vi "Receiver_Example_Img - Copy (2).vi"() -> ()   [LabVIEW 2018]
uses:
  <vilib>/picture/picture.llb/imagedata.ctl
panel:
  in  "path to BMP file":path=path "D:/Thesis Pak Pri/pict.bmp"
  out "Constellation Diagram Receiver":cdb[](graph)
  out "0, 2":i16[][](array[numeric])
  out "1-bit pixmap   2":bool[][](array[boolean])
  out "new picture 2":picture
  out "image data 2":T1
  in  "Image File Reference":path=path "D:/Thesis Pak Pri/boo.bmp"
  out "Array":i32[](array[numeric])
  out "x/y 3":dbl
  out "size bit output":i32
  out "BER":dbl
  out "Numeric":i32
  out "bit output":i32[][](array[numeric])
  out "output diterima":bool[][](array[boolean])
  out "Output Image":picture
  in  "Width":i32=256
  in  "Height":i32=256
  out "x/y":dbl
  out "x > y?":bool
  out "size(s)":i32
  out "bit received":i8[](array[numeric])
  in  "Bit length (set)":i32=3600
  out "sisa bagi":i32
  out "hasil bagi":i32
  out "iterasi":i32
  in  "Modulation parameter":T2
  out "created new?":bool
  out "SIG valid?":bool
  in  "stop":bool
  out "USRP CoercedParamters":T3={"coerced IQ rate"=100000.0, "coerced carrier frequency"=100000.0, "coerced gain"=0.0} {"coerced gain" format="%#_6f"; "coerced carrier frequency" format="%#_6p"; "coerced IQ rate" format="%#_6p"}
  out "error out":errorcluster
  in  "Trigger level":dbl=0.005 format="%f"
  in  "error in (no error)":errorcluster
  in  "USRP ControledParameters":T4={"active antenna"="RX1", "gain"=0.0, "carrier frequency"=915000000.0, "IQ rate"=1000000.0} {"IQ rate" format="%#_6p"; "carrier frequency" format="%#_6p"; "gain" format="%#_6f"}
  in  "device names":refnum<k15>="192.168.10.4"
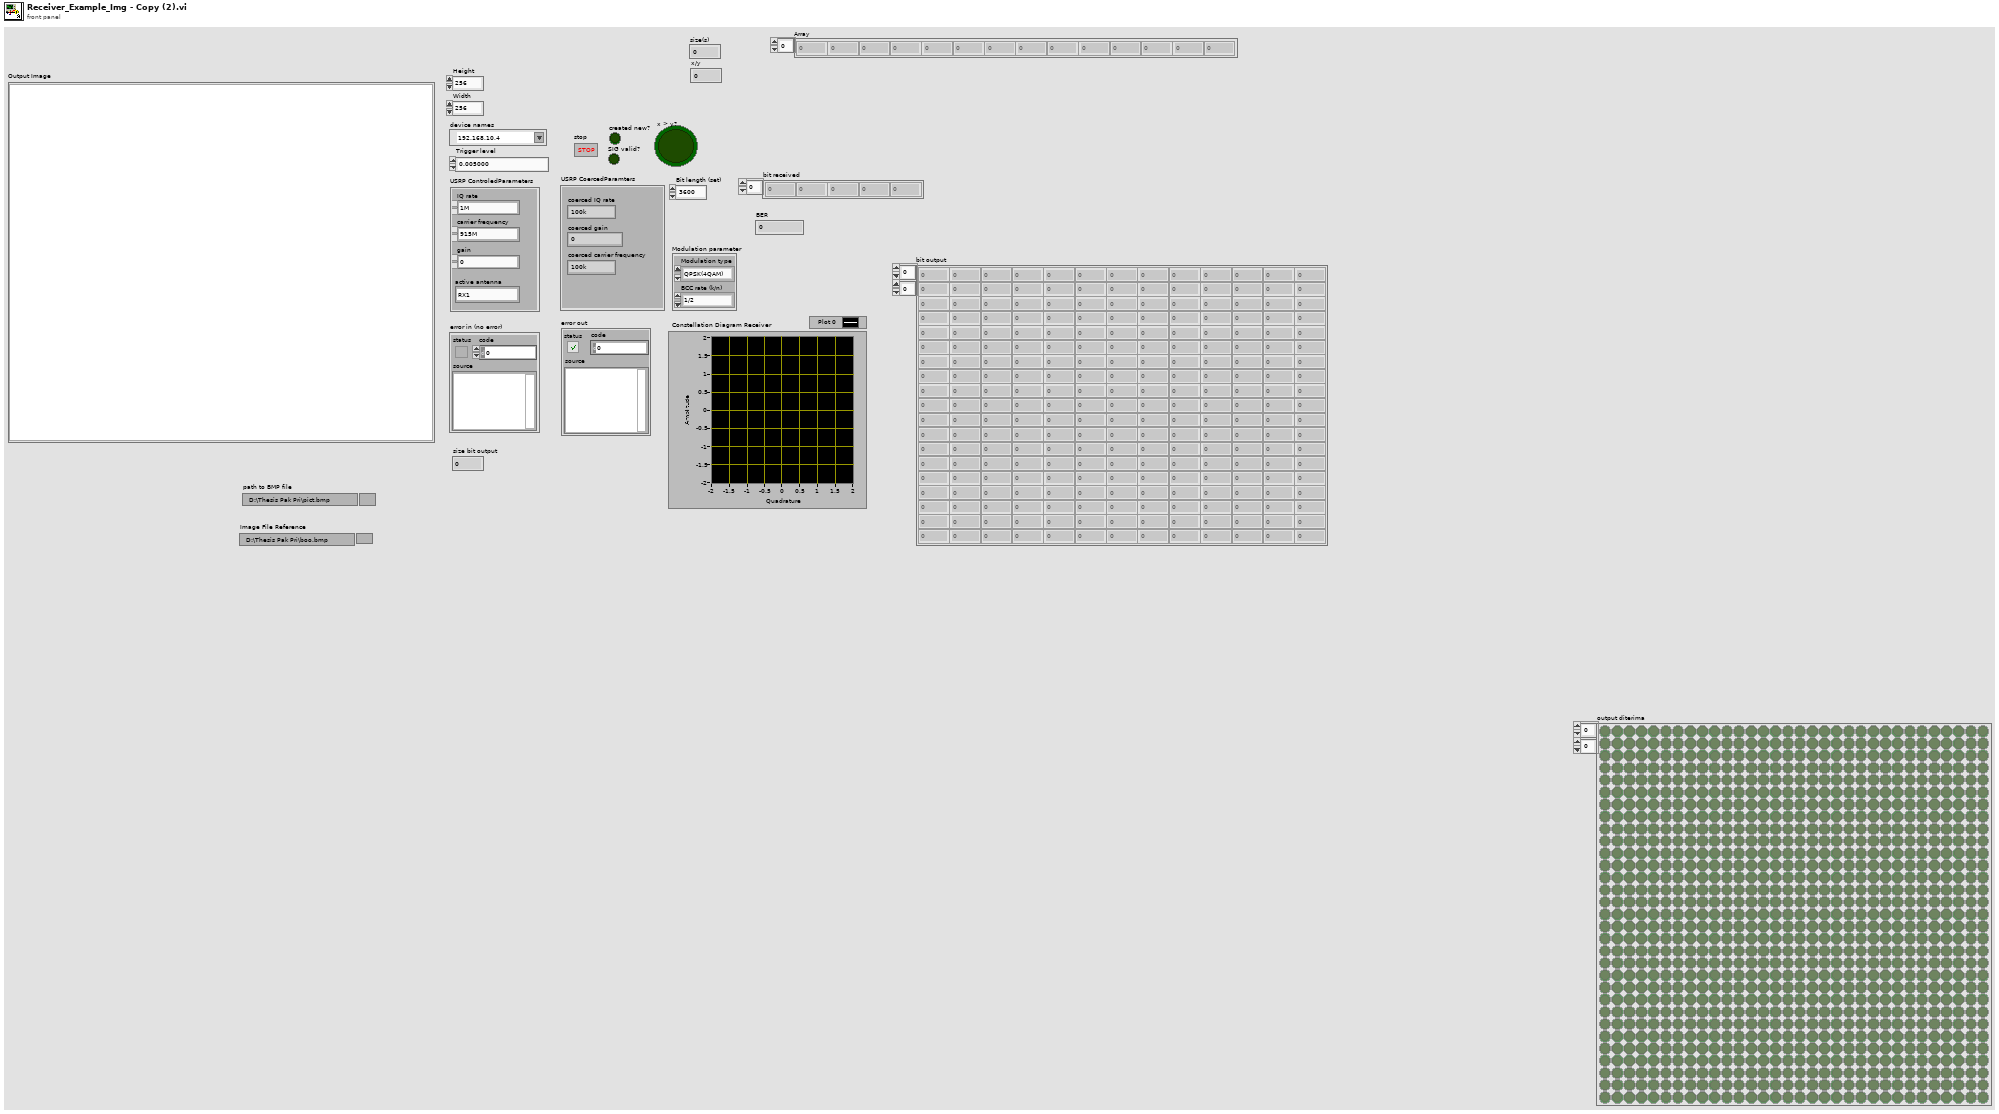
[diagram p1: front panel]
types:
  T1 = typedef "imagedata.ctl" = cluster{"image type":i32, "image depth":i32, "image":u8[], "mask":u8[], "colors":u32[], "Rectangle":cluster{"left":i16, "top":i16, "right":i16, "bottom":i16}}
  T2 = cluster{"Modulation type":enum16{"QPSK(4QAM)", "64QAM", "16QAM", "BPSK"}, "BCC rate (k/n)":enum16{"1/2", "2/3", "3/4"}}
  T3 = cluster{"coerced IQ rate":dbl, "coerced carrier frequency":dbl, "coerced gain":dbl}
  T4 = cluster{"active antenna":string, "gain":dbl, "carrier frequency":dbl, "IQ rate":dbl}
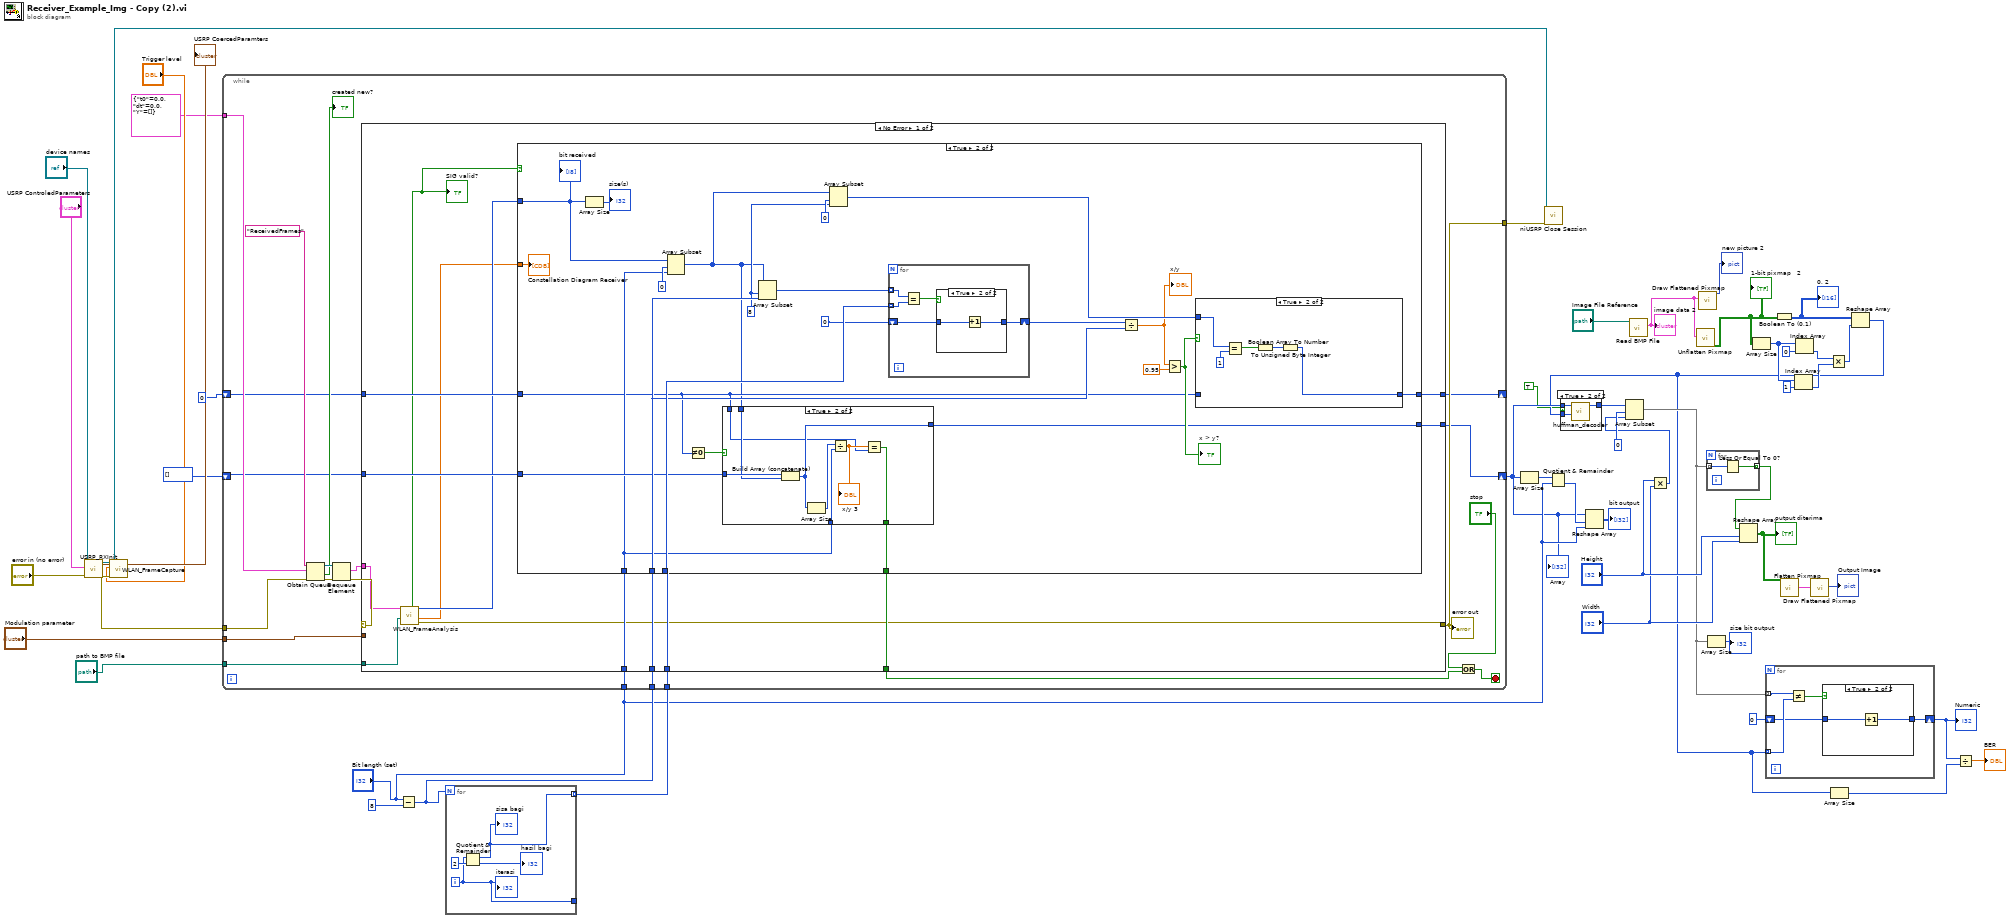
[diagram p0: block diagram]
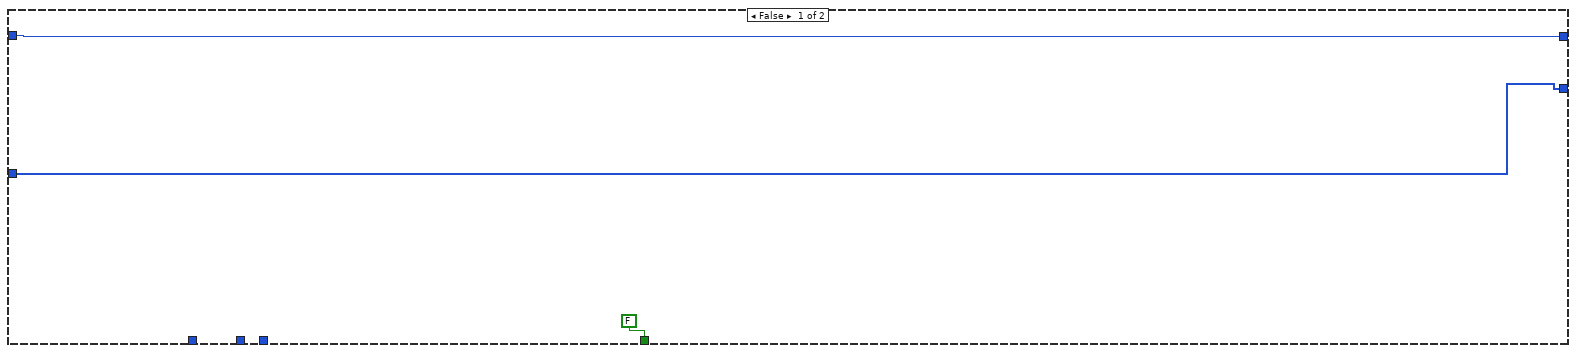
[diagram p4: hidden frame]
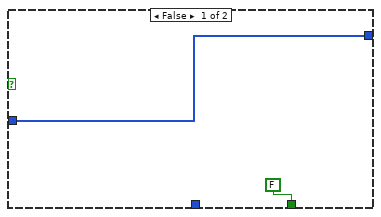
[diagram p5: hidden frame]
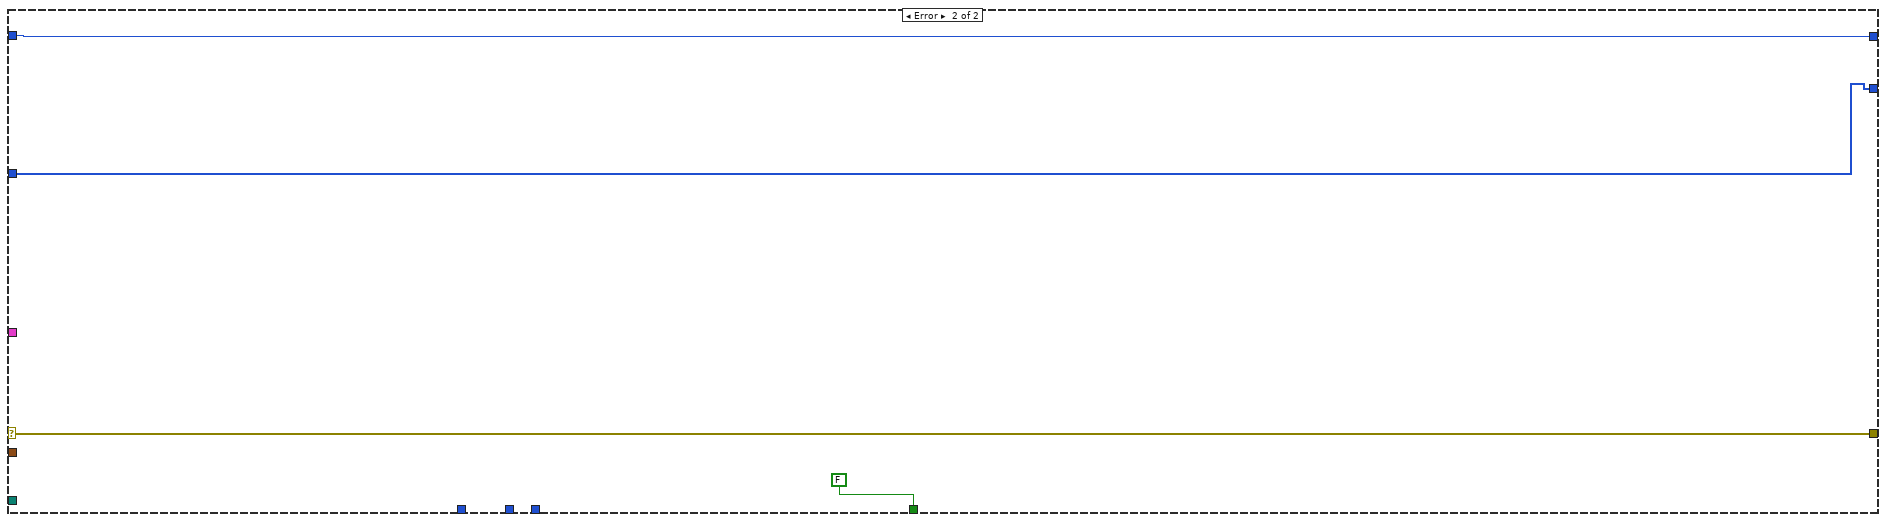
[diagram p8: hidden frame]
diagram:
  n1 = call "USRP_RXInit.vi"("device names"="device names", "USRP ControledParameters"="USRP ControledParameters", "error in (no error)"="error in (no error)") -> ("session handle out"=w41:refnum<k15>, "USRP CoercedParamters"=→"USRP CoercedParamters":T3, "error out"=w45:errorcluster)  [unwired: 5 in]
  n2 = call "WLAN_FrameCapture.vi"("error in (no error)"=w45, "Trigger level"="Trigger level", "session handle"=w41) -> ()  [unwired: 8 in]
  n3 = Subtract(x="Bit length (set)", y=8) -> (x-y=w38:i32)
  n4 = for {
    N: w38 -> [_]
    tunnel: [w51] -> _
    tunnel: [w50] -> w37 mode=indexing
    i -> [w51]
    n5 = Quotient & Remainder(x=w51, y=2) -> (x-y*floor(x/y)=w50:i32, floor(x/y)=→"hasil bagi":i32)
    "sisa bagi" <- w50
    "iterasi" <- w51
  }
  n6 = while {
    tunnel: w45 -> [w73]
    tunnel: cluster{"t0":dbl, "dt":dbl, "Y":cdb[]} {"t0"=0.0, "dt"=0.0, "Y"=[]} ("data") -> [w74]
    tunnel: [w66] -> w42
    tunnel: "Modulation parameter" -> [w65]
    tunnel: "Bit length (set)" -> [w64]
    tunnel: w38 -> [w63]
    tunnel: w37 -> [w62]
    shift-right: [w60] -> _
    shift-left: 0 -> [w61]
    shift-right: [w58] -> w6
    shift-left: i32[] [] -> [w59]
    tunnel: "path to BMP file" -> [w54]
    stop <- w55 stop-if-true
    n7 = Obtain Queue(name (unnamed)="ReceivedFrames", element data type=w74, error in (no error)=w73) -> (queue out=w72:refnum<queue>, created new?=→"created new?":bool, error out=w69:errorcluster)  [unwired: 2 in]
    n8 = Dequeue Element(queue=w72, error in (no error)=w69) -> (element=w70:cluster{"t0":dbl, "dt":dbl, "Y":cdb[]}, error out=w71:errorcluster)  [unwired: 1 in, 2 out]
    n9 = case shown="No Error" w71 {
      selector: w71 -> [_ w142]
      tunnel: w70 -> [w80 _]
      tunnel: [w79 w142] -> w66
      tunnel: w65 -> [_ _]
      tunnel: w64 -> [w88 _]
      tunnel: w63 -> [w87 _]
      tunnel: w62 -> [w86 _]
      tunnel: w61 -> [w85 w141]
      tunnel: [w84 w141] -> w60
      tunnel: w59 -> [w83 w140]
      tunnel: [w82 w140] -> w58
      tunnel: [w81 FALSE] -> w56
      tunnel: w54 -> [w75 _]
      frame No Error {
        n10 = call "WLAN_FrameAnalysis.vi"("path to BMP file"=w75, "input cluster"=w80) -> ("error out"=w79:errorcluster, "Constellation"=w76:cdb[], "output bits"=w77:i8[], "SIG valid?"=w78:bool)  [unwired: 3 in, 3 out]
        "SIG valid?" <- w78
        n11 = case shown="True" w78 {
          tunnel: w77 -> [_ w93]
          tunnel: w76 -> [_ w92]
          tunnel: w88 -> [_ w99]
          tunnel: w87 -> [_ w108]
          tunnel: w86 -> [_ w111]
          tunnel: w85 -> [w91 w98]
          tunnel: [w91 w102] -> w84
          tunnel: w83 -> [w90 w100]
          tunnel: [w90 w96] -> w82
          tunnel: [FALSE w97] -> w81
          frame False {
          }
          frame True {
            w104 = 8 ("index")
            n12 = Array Size(array=w93) -> (size(s)=→"size(s)":i32)
            n13 = Array Subset(array=w93, index=0, length=w99) -> (w94:i8[])
            n14 = Not Equal To 0?(x=w98) -> (x != 0?=w101:bool)
            n15 = case shown="True" w101 {
              tunnel: w100 -> [w116 w124]
              tunnel: w94 -> [_ w123]
              tunnel: [w116 w120] -> w96
              tunnel: w99 -> [_ w119]
              tunnel: w98 -> [_ w118]
              tunnel: [FALSE w117] -> w97
              frame False {
              }
              frame True {
                n16 = Build Array (concatenate)(w124, w123) -> (w120:i32[])
                n17 = Array Size(array=w120) -> (size(s)=w122:i32)
                n18 = Divide(x=w122, y=w119) -> (x/y=w121:dbl)
                "x/y 3" <- w121
                n19 = Equal?(x=w121, y=w118) -> (x = y?=w117:bool)
              }
            }
            n20 = Array Subset(array=w94, index=w104, length=w108) -> (w112:i8[])
            n21 = Array Subset(array=w94, index=0, length=w104) -> (w103:i8[])
            n22 = for {
              tunnel: w112 -> [w134] mode=indexing
              tunnel: w111 -> [w135] mode=indexing
              shift-right: [w131] -> w109
              shift-left: 0 -> [w132]
              n23 = Equal?(x=w134, y=w135) -> (x = y?=w133:bool)
              n24 = case shown="True" w133 {
                tunnel: w132 -> [w136 w138]
                tunnel: [w136 w137] -> w131
                frame False {
                }
                frame True {
                  n25 = Increment(x=w138) -> (x+1=w137:i32)
                }
              }
            }
            n26 = Divide(x=w109, y=w108) -> (x/y=w95:dbl)
            "x/y" <- w95
            n27 = Greater?(x=w95, y=0.95) -> (0:w106:bool)
            "x > y?" <- w106
            n28 = case shown="True" w106 {
              tunnel: w103 -> [_ w128]
              tunnel: w98 -> [w125 _]
              tunnel: [w125 w126] -> w102
              frame False {
              }
              frame True {
                n29 = Equal?(x=w128, y=1) -> (x = y?=w129:bool[])
                n30 = Boolean Array To Number(Boolean array=w129) -> (number=w127:u32)
                n31 = To Unsigned Byte Integer(number=w127) -> (unsigned 8bit integer=w126:u8)
              }
            }
            "bit received" <- w93
            "Constellation Diagram Receiver" <- w92
          }
        }
      }
      frame Error {
      }
    }
    "error out" <- w66
    n32 = Or(x="stop", y=w56) -> (x .or. y?=w55:bool)
  }
  "Array" <- w6
  n33 = Array Size(array=w6) -> (size(s)=w34:i32)
  n34 = call <instrlib>:"niUSRP Close Session.vi"("session handle"=w41, "error in (no error)"=w42) -> ()  [unwired: 13 in, 1 out]
  n35 = Quotient & Remainder(x=w34, y="Bit length (set)") -> (floor(x/y)=w26:i32)  [unwired: 1 out]
  n36 = Reshape Array(w6, w26, "Bit length (set)") -> (→"bit output":i32[][])
  n37 = call <vilib>:"Read BMP File.vi"("path to BMP file"="Image File Reference") -> ("image data"=w15:T1)  [unwired: 8 in, 2 out]
  "image data 2" <- w15
  n38 = Multiply(x="Height", y="Width") -> (x*y=w27:i32)
  n39 = call <vilib>:"Unflatten Pixmap.vi"("image data"=w15) -> ("1-bit pixmap"=w13:bool[][])  [unwired: 4 in, 6 out]
  "1-bit pixmap   2" <- w13
  n40 = call <vilib>:"Draw Flattened Pixmap.vi"("image data"=w15) -> ("new picture"=→"new picture 2":picture)  [unwired: 8 in]
  n41 = Array Size(array=w13) -> (size(s)=w10:i32[])
  n42 = Boolean To (0,1)(Boolean=w13) -> (0, 1=w14:i16[][])
  "0, 2" <- w14
  n43 = Index Array(array=w10, index=1) -> (element=w8:i32)
  n44 = Index Array(array=w10, index=0) -> (element=w9:i32)
  n45 = Multiply(x=w9, y=w8) -> (x*y=w7:i32)
  n46 = Reshape Array(w14, w7) -> (w3:i16[])
  n47 = case shown="True" TRUE {
    tunnel: w6 -> [w143 w146]
    tunnel: [w143 w145] -> w5
    tunnel: w3 -> [_ w144]
    frame False {
    }
    frame True {
      n48 = call "huffman_decoder.vi"("data_array_bit"=w144, "encode_array_bit"=w146) -> ("return value"=w145:i32[])  [unwired: 9 in]
    }
  }
  n49 = Array Subset(array=w5, index=0, length=w27) -> (w4:i32[])
  n50 = for {
    tunnel: w4 -> [w148] mode=indexing
    tunnel: [w147] -> w32 mode=indexing
    n51 = Less Or Equal To 0?(x=w148) -> (x <= 0?=w147:bool)
  }
  n52 = Array Size(array=w4) -> (size(s)=→"size bit output":i32)
  n53 = Reshape Array(w32, "Height", "Width") -> (w31:bool[][])
  "output diterima" <- w31
  n54 = for {
    tunnel: w4 -> [w153] mode=indexing
    tunnel: w3 -> [w152] mode=indexing
    shift-right: [w149] -> w22
    shift-left: 0 -> [w150]
    n55 = Not Equal?(x=w153, y=w152) -> (x != y?=w151:bool)
    n56 = case shown="True" w151 {
      tunnel: w150 -> [w154 w156]
      tunnel: [w154 w155] -> w149
      frame False {
      }
      frame True {
        n57 = Increment(x=w156) -> (x+1=w155:i32)
      }
    }
  }
  "Numeric" <- w22
  n58 = call <vilib>:"Flatten Pixmap.vi"("1-bit pixmap"=w31) -> ("image data"=w33:T1)  [unwired: 10 in]
  n59 = call <vilib>:"Draw Flattened Pixmap.vi"("image data"=w33) -> ("new picture"=→"Output Image":picture)  [unwired: 8 in]
  n60 = Array Size(array=w3) -> (size(s)=w21:i32)
  n61 = Divide(x=w22, y=w21) -> (x/y=→"BER":dbl)
